vi "Write Local IP Address.vi"(10 "Local IP":string, 11 "TCP Stream Listener in":refnum<class "TCP Stream Listener.lvclass">) -> (3 "TCP Stream Listener out":refnum<class "TCP Stream Listener.lvclass">)   [LabVIEW 2020, in "TCP Stream Listener.lvclass"]
doc: "Use this accessor to specify the local IP address the listener endpoint should use, should more than one NIC be available. You do not need, and should not use, this accessor if only one NIC is available."
uses:
  TCP Stream Listener.lvclass
  TCP Stream Listener.lvclass/TCP Stream Listener.ctl
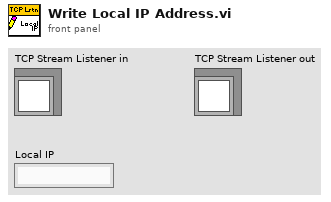
[diagram p1: front panel]
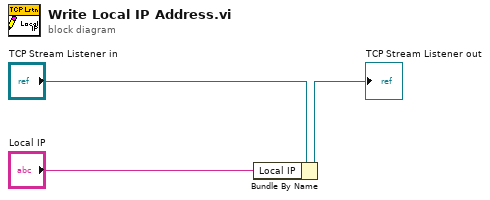
[diagram p0: block diagram]
diagram:
  n1 = Bundle By Name(cluster="TCP Stream Listener in", "Local IP"="Local IP") -> (→"TCP Stream Listener out":refnum<class "TCP Stream Listener.lvclass">)
